vi "Elevator Controller.vi"(8 "error in":errorcluster) -> ()   [LabVIEW 2017]
doc: "This VI executes continuously carrying out the current operation and responding to updates or new operations. It will often contain the timing or control code that is difficult to place directly in TeleOp. This VI generally opens all sensors and motors and isolates the rest of the robot code from knowing how the operations are carried out."
uses:
  <vilib>/Rock Robotics/WPI/Framework/Completion Status.ctl
  Elevator Setpoints.ctl
  Elevator Operations.ctl
  <vilib>/Rock Robotics/WPI/Solenoid/WPI_SolenoidChannel.ctl
  <vilib>/Rock Robotics/WPI/ThirdParty/Phoenix-LabVIEW/Motor Controller/Controls/CTRE_Phoenix_MotorControl_FeedbackDevice.ctl
  <vilib>/Rock Robotics/SystemInterfaces/DIO/FPGA_DIOChannel.ctl
  <vilib>/Rock Robotics/WPI/SafetyOutput/WPI_SafetyOutputConfigMenu.ctl
  <vilib>/Rock Robotics/WPI/ThirdParty/Phoenix-LabVIEW/Motor Controller/Controls/CTRE_Phoenix_MotorControl_NeutralMode.ctl
  <vilib>/Rock Robotics/WPI/ThirdParty/Phoenix-LabVIEW/Motor Controller/Controls/CTRE_Phoenix_MotorControl_ControlMode.ctl
  <vilib>/Rock Robotics/WPI/Solenoid/WPI_SolenoidValue.ctl
  <vilib>/Rock Robotics/WPI/Solenoid/WPI_SolenoidOpenDouble.vi
  <vilib>/Rock Robotics/WPI/Switch/WPI_SwitchOpenLimit.vi
  Elevator Published Globals.vi
  <vilib>/Rock Robotics/WPI/Solenoid/WPI_SolenoidSetEnum.vi
  <vilib>/Rock Robotics/Network Tables/NT Write Boolean.vi
panel:
  in  "Interactive Values":T1
  out "Current\nCmd":string
  in  "Buttons":cluster{"Execute Cmd":bool, "Abort Cmd":bool}
  out "Command Timing":cluster{"Start Time (ms)":u32, "Iterations":i32}
  out "Status":T3
  # "Tip: It may be helpful to observe inputs and sensor values.\nYou may also want to display tuning or debugging controls."
  # "Interactive Command: You may fill in the settings for a command\nand schedule it with the Execute button. You can observe and abort\nany command while fine tuning the code for the controller."
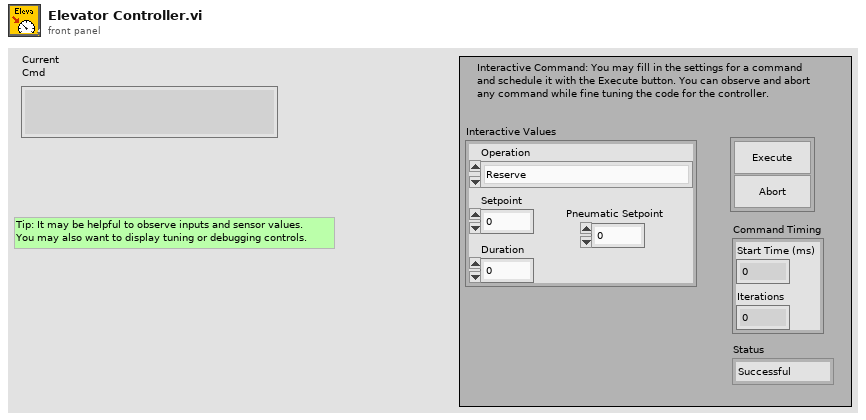
[diagram p1: front panel]
types:
  T1 = typedef "Elevator Setpoints.ctl" = cluster{"Operation":T2, "Setpoint":dbl, "Duration":dbl, "Pneumatic Setpoint":dbl}
  T2 = typedef "Elevator Operations.ctl" = enum16{"Reserve", "Read Current", "Pick Up Cube (Lowest)", "Switch", "Scale", "Immediate"}
  T3 = typedef "Completion Status.ctl" = enum16{"Successful", "Aborted", "Incomplete"}
  T4 = typedef "CTRE_Phoenix_MotorControl_NeutralMode.ctl" = enum8{"EEPROMSetting", "Override to Coast", "Override to Brake"}
  T5 = typedef "WPI_SafetyOutputConfigMenu.ctl" = enum16{"Enable", "Disable"}
  T6 = typedef "FPGA_DIOChannel.ctl" = enum8{"DIO 0", "DIO 1", "DIO 2", "DIO 3", "DIO 4", "DIO 5", "DIO 6", "DIO 7", "DIO 8", "DIO 9", "DIO MXP 0", "DIO MXP 1", "DIO MXP 2", "DIO MXP 3", "DIO MXP 4", "DIO MXP 5", "DIO MXP 6", "DIO MXP 7", "DIO MXP 8", "DIO MXP 9", "DIO MXP 10", "DIO MXP 11", "DIO MXP 12", "DIO MXP 13", "DIO MXP 14", "DIO MXP 15", "SPI Port CS1", "SPI Port CS2", "SPI Port CS3", "SPI Port MISO", "SPI Port MOSI", "Invalid"}
  T7 = typedef "CTRE_Phoenix_MotorControl_FeedbackDevice.ctl" = i8
  T8 = typedef "WPI_SolenoidChannel.ctl" = enum8{"Solenoid 0", "Solenoid 1", "Solenoid 2", "Solenoid 3", "Solenoid 4", "Solenoid 5", "Solenoid 6", "Solenoid 7", "Invalid"}
  T9 = typedef "WPI_MotorControlDeviceRef.ctl" = cluster{"DeviceStatus":errorcluster, "Type":T10, "PWM":cluster{"PWM Channel":T11, "DeadBand":T12}, "CAN":cluster{"Device Number":u8, "SetOutput VI Ref":variant, "GetOutput VI Ref":variant, "Enable VI Ref":variant, "Disable VI Ref":variant, "Data":variant}, "Invert":bool, "DIO PWM":cluster{"PWM \"Enable\" Channel":T11, "DIOChannel":T6, "PWM Rate":dbl}}
  T10 = typedef "WPI_MotorControlType.ctl" = enum16{"PWM", "CAN", "DIO PWM"}
  T11 = typedef "FPGA_DIOPWMChannel.ctl" = enum8{"PWM 0", "PWM 1", "PWM 2", "PWM 3", "PWM 4", "PWM 5", "PWM 6", "PWM 7", "PWM 8", "PWM 9", "PWM MXP 0", "PWM MXP 1", "PWM MXP 2", "PWM MXP 3", "PWM MXP 4", "PWM MXP 5", "PWM MXP 6", "PWM MXP 7", "PWM MXP 8", "PWM MXP 9", "Invalid"}
  T12 = typedef "WPI_PWMDeadband.ctl" = cluster{"Name":string, "maxPositivePwm":i32, "minPositivePwm":i32, "centerPwm":i32, "maxNegativePwm":i32, "minNegativePwm":i32, "angularRange":u16}
  T13 = typedef "WPI_SolenoidDevRef.ctl" = cluster{"DevStatus":errorcluster, "Pneumatics Control Module":u8, "Forward Solenoid Channel":T8, "Reverse Solenoid Channel":T8}
  T14 = typedef "WPI_SwitchDevRef.ctl" = cluster{"DevStatus":errorcluster, "DIO Channel":T6, "CntIndex":T15, "Normally Closed":bool}
  T15 = typedef "FPGA_CounterCtrSystemIndex.ctl" = enum8{"Ctr 0", "Ctr 1", "Ctr 2", "Ctr 3", "Ctr 4", "Ctr 5", "Ctr 6", "Ctr 7", "Invalid"}
  T16 = typedef "Command Status Info.ctl" = cluster{"Name":string, "Status":T3, "notifier out":T17}
  T17 = typedef "Completion Notifier.ctl" = refnum<notifier>
  T18 = cluster{"Current Command":T1, "Command Timing":cluster{"Start Time (ms)":u32, "Iterations":i32}, "Command Arguments":cluster{"Command Info":T16, "Description":string, "Default Command":T1, "queue out":refnum<queue>, "Subsystem Name":string}}
  T19 = typedef "WPI_SolenoidValue.ctl" = enum16{"Off", "On", "Forward", "Reverse"}
  T20 = typedef "CTRE_Phoenix_MotorControl_ControlMode.ctl" = u16
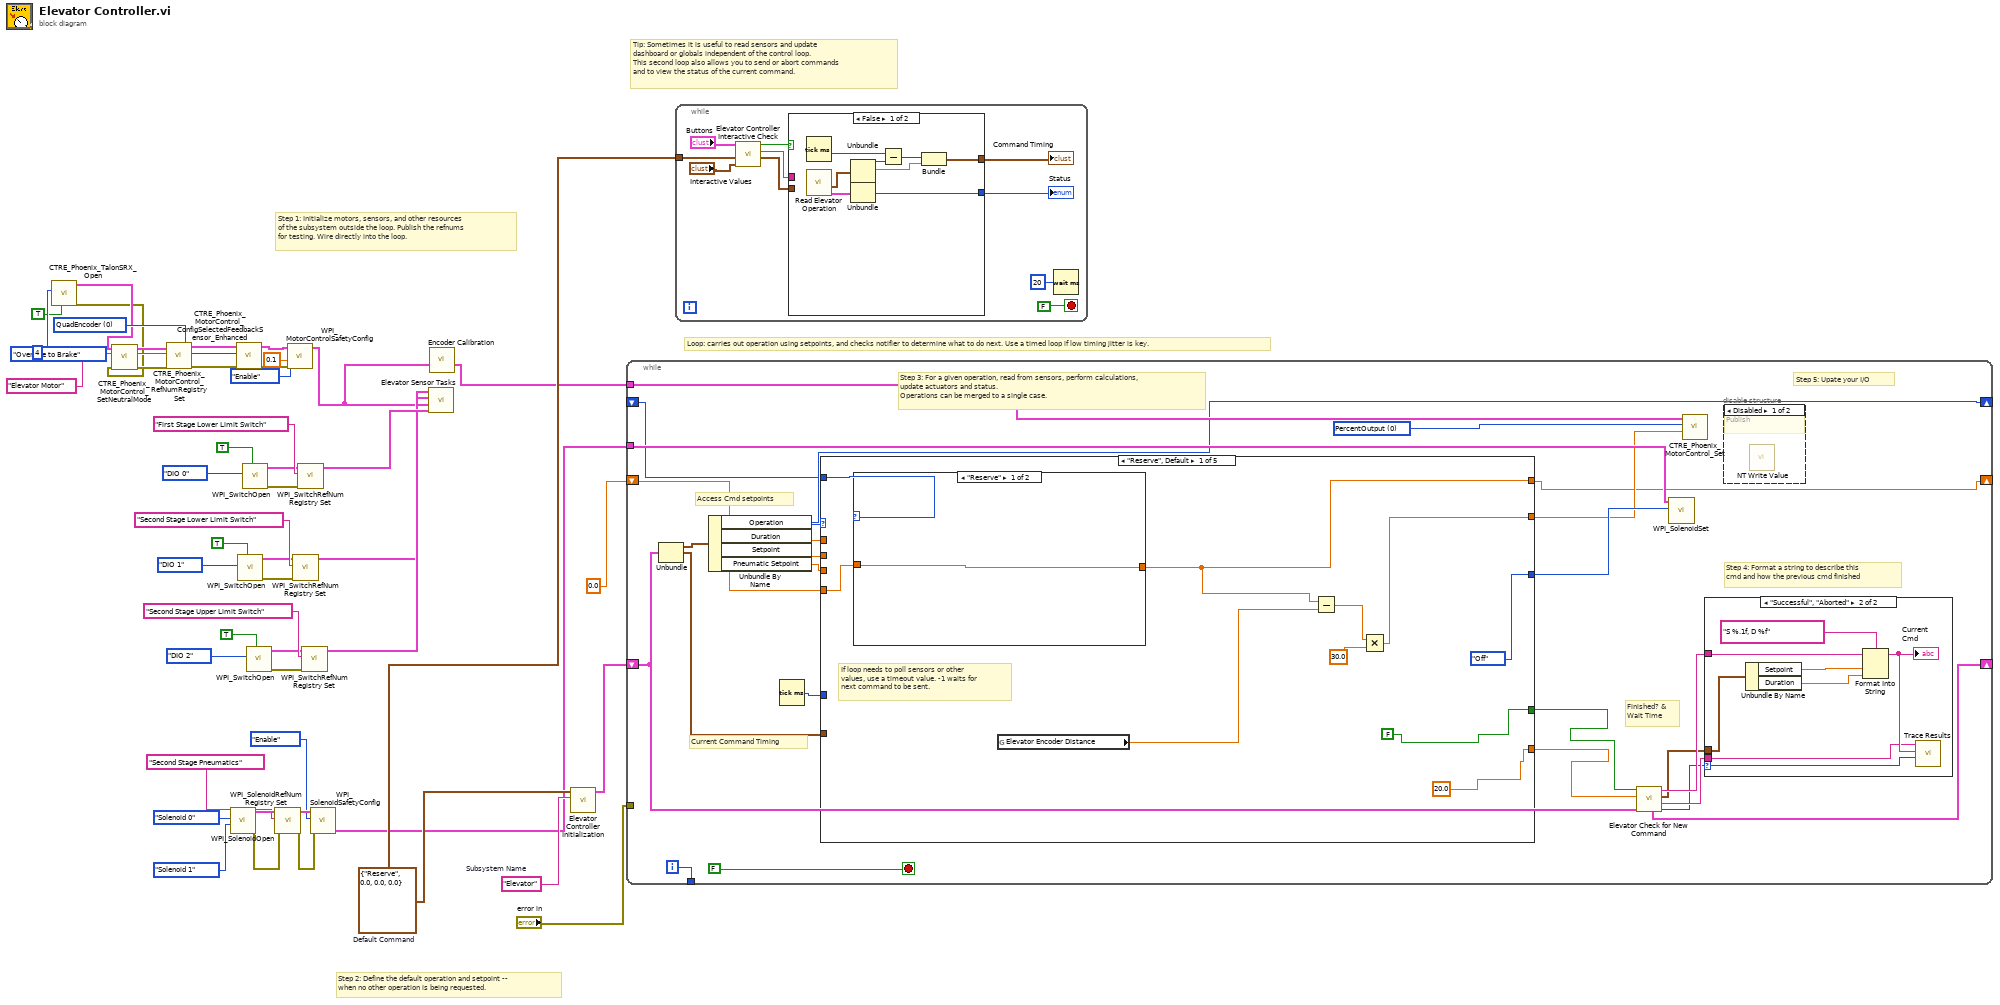
[diagram p0: block diagram]
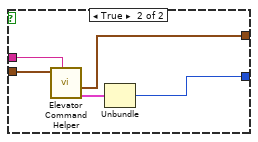
[diagram p2: hidden frame]
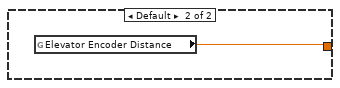
[diagram p5: hidden frame]
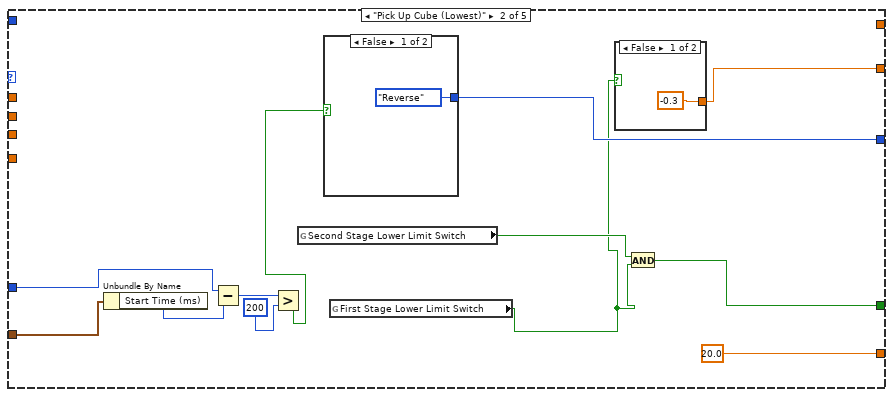
[diagram p6: hidden frame]
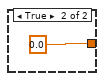
[diagram p7: hidden frame]
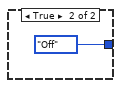
[diagram p8: hidden frame]
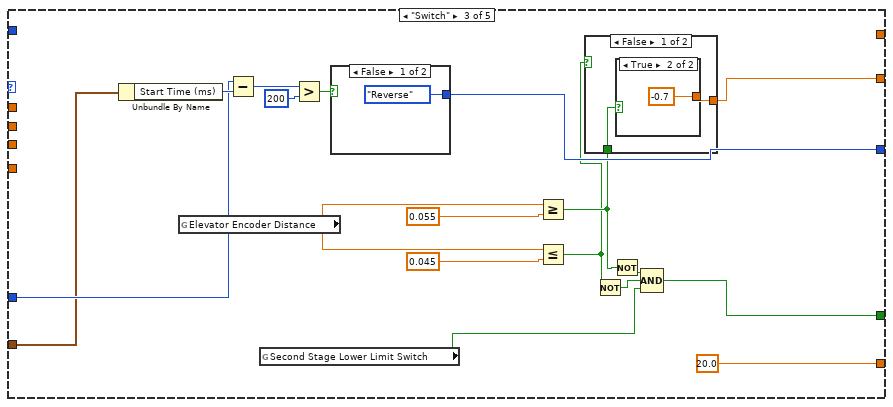
[diagram p9: hidden frame]
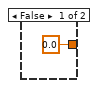
[diagram p10: hidden frame]
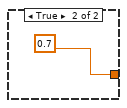
[diagram p11: hidden frame]
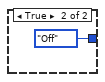
[diagram p12: hidden frame]
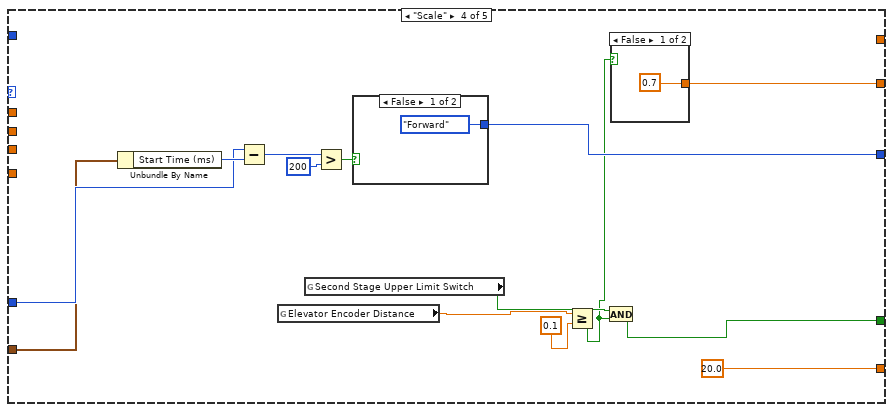
[diagram p13: hidden frame]
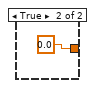
[diagram p14: hidden frame]
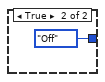
[diagram p15: hidden frame]
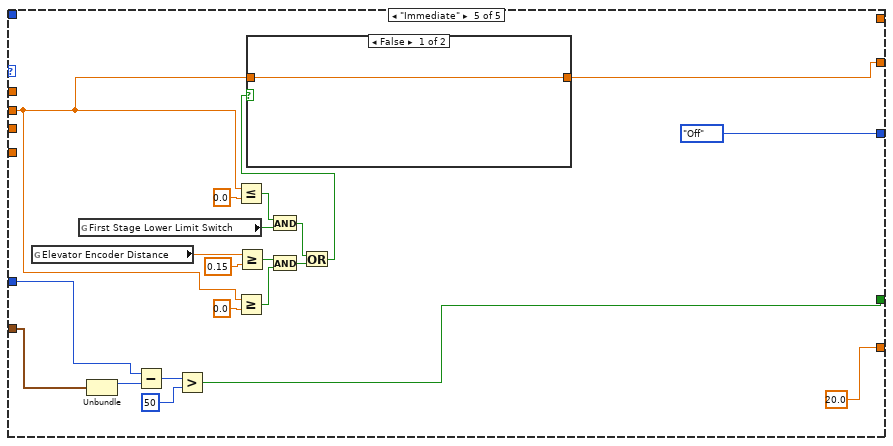
[diagram p16: hidden frame]
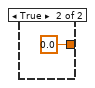
[diagram p17: hidden frame]
diagram:
  w33 = T7 0 items=["None"=-1, "QuadEncoder"=0, "Analog"=2, "Tachometer"=4, "Pulse Width Encoded Position"=8, "Sensor Sum (S0 + S1)"=9, "Sensor Difference (D0 - D1)"=10, "Remote Source 0"=11, "Remote Source 1"=12, "Software Emulated"=15] ("Feedback Device")
  w46 = T1 {"Operation"=enum."Reserve", "Setpoint"=0.0, "Duration"=0.0, "Pneumatic Setpoint"=0.0}  # Default Command
  w47 = "Elevator"  # Subsystem Name
  # "Tip: Sometimes it is useful to read sensors and update\ndashboard or globals independent of the control loop.\nThis second loop also allows you to send or abort commands\nand to view the status of the current command."
  # "Step 2: Define the default operation and setpoint --\nwhen no other operation is being requested."
  # "Step 1: Initialize motors, sensors, and other resources\nof the subsystem outside the loop. Publish the refnums\nfor testing. Wire directly into the loop."
  # "Loop: carries out operation using setpoints, and checks notifier to determine what to do next. Use a timed loop if low timing jitter is key."
  n1 = call <vilib>:"CTRE_Phoenix_TalonSRX_Open.vi"("Invert"=TRUE, "Device Number"=u8 4) -> ("error out"=w22:errorcluster, "CAN Talon SRX Ref"=w25:T9)  [unwired: 8 in]
  n2 = call <vilib>:"CTRE_Phoenix_MotorControl_SetNeutralMode.vi"("error in (no error)"=w22, "Motor Control Neutral Mode"=CTRE_Phoenix_MotorControl_NeutralMode."Override to Brake", "PhoenixMotorControlDevRef"=w25) -> ("error out"=w23:errorcluster, "PhoenixMotorControlDevRef"=w24:T9)  [unwired: 7 in]
  n3 = call <vilib>:"CTRE_Phoenix_MotorControl_RefNumRegistrySet.vi"("error in (no error)"=w23, "refnum name"="Elevator Motor", "PhoenixMotorControlDevRef"=w24) -> ("error out"=w32:errorcluster, "PhoenixMotorControlDevRef"=w34:T9)  [unwired: 7 in]
  n4 = call-poly <vilib>:"WPI_SolenoidOpen.vi"("Reverse Solenoid Channel"=WPI_SolenoidChannel."Solenoid 1", "Forward Solenoid Channel"=WPI_SolenoidChannel."Solenoid 0") -> ("error out"=w42:errorcluster, "SolenoidDevRef"=w43:T13)  [unwired: 8 in]
  n5 = call <vilib>:"CTRE_Phoenix_MotorControl_ConfigSelectedFeedbackSensor_Enhanced.vi"("error in (no error)"=w32, "Feedback Device"=w33, "PhoenixMotorControlDevRef"=w34) -> ("error out"=w5:errorcluster, "PhoenixMotorControlDevRef"=w7:T9)  [unwired: 7 in]
  n6 = call-poly <vilib>:"WPI_SwitchOpen.vi"("Normally Closed"=TRUE, "DIO Channel"=FPGA_DIOChannel."DIO 1") -> ("error out"=w19:errorcluster, "SwitchDevRef"=w17:T14)  [unwired: 8 in]
  n7 = call-poly <vilib>:"WPI_SwitchOpen.vi"("Normally Closed"=TRUE, "DIO Channel"=FPGA_DIOChannel."DIO 0") -> ("error out"=w29:errorcluster, "SwitchDevRef"=w27:T14)  [unwired: 8 in]
  n8 = call-poly <vilib>:"WPI_SwitchOpen.vi"("Normally Closed"=TRUE, "DIO Channel"=FPGA_DIOChannel."DIO 2") -> ("error out"=w14:errorcluster, "SwitchDevRef"=w12:T14)  [unwired: 8 in]
  n9 = call <vilib>:"WPI_SolenoidRefNum Registry Set.vi"("error in (no error)"=w42, "refnum name"="Second Stage Pneumatics", "SolenoidDevRef"=w43) -> ("error out"=w41:errorcluster, "SolenoidDevRef"=w44:T13)  [unwired: 7 in]
  n10 = call <vilib>:"WPI_MotorControlSafetyConfig.vi"("error in (no error)"=w5, "timeout (s)"=0.1, "mode"=WPI_SafetyOutputConfigMenu."Enable", "MotorControlDevRef"=w7) -> ("MotorControlDevRef"=w6:T9)  [unwired: 6 in, 1 out]
  n11 = call <vilib>:"WPI_SwitchRefNum Registry Set.vi"("error in (no error)"=w19, "refnum name"="Second Stage Lower Limit Switch", "SwitchDevRef"=w17) -> ("SwitchDevRef"=w10:T14)  [unwired: 7 in, 1 out]
  n12 = call <vilib>:"WPI_SwitchRefNum Registry Set.vi"("error in (no error)"=w29, "refnum name"="First Stage Lower Limit Switch", "SwitchDevRef"=w27) -> ("SwitchDevRef"=w26:T14)  [unwired: 7 in, 1 out]
  n13 = call <vilib>:"WPI_SwitchRefNum Registry Set.vi"("error in (no error)"=w14, "refnum name"="Second Stage Upper Limit Switch", "SwitchDevRef"=w12) -> ("SwitchDevRef"=w11:T14)  [unwired: 7 in, 1 out]
  n14 = call <vilib>:"WPI_SolenoidSafetyConfig.vi"("error in (no error)"=w41, "mode"=WPI_SafetyOutputConfigMenu."Enable", "SolenoidDevRef"=w44) -> ("SolenoidDevRef"=w45:T13)  [unwired: 7 in, 1 out]
  n15 = call "Elevator Sensor Tasks.vi"("SecondUpperElevatorSwitchDevRef"=w11, "SecondLowerElevatorSwitchDevRef"=w10, "ElevatorControllerDevRef"=w6, "FirstLowerElevatorSwitchDevRef"=w26) -> ()  [unwired: 7 in]
  n16 = call "Encoder Calibration.vi"("PhoenixMotorControlDevRef"=w6) -> ("PhoenixMotorControlDevRef Out"=w9:T9)  [unwired: 10 in]
  n17 = call "Elevator Controller Initialization.vi"("Subsystem Name"=w47, "Default Command"=w46) -> ("Current Command"=w48:T18)  [unwired: 9 in]
  n18 = while {
    shift-right: [w67] -> _
    shift-left: w48 -> [w60]
    tunnel: [w73] -> _
    tunnel: "error in" -> [_]
    tunnel: w45 -> [w59]
    tunnel: w9 -> [w57]
    shift-right: [w53] -> _
    shift-left: _ -> [w52]
    shift-right: [w51] -> _
    shift-left: 0.0 -> [w50]
    i -> [w73]
    stop <- FALSE stop-if-true
    w56 = T20 0 items=["PercentOutput"=0, "Position"=1, "Velocity"=2, "Current"=3, "Follower"=5, "MotionProfile"=6, "MotionMagic"=7, "MotionMagicArc"=8, "MotionProfileArc"=10, "Disabled"=15] ("Control Mode")
    # "Step 5: Upate your I/O"
    # "Step 4: Format a string to describe this\ncmd and how the previous cmd finished"
    # "Current Command Timing"
    # "Access Cmd setpoints"
    # "Finished? &\nWait Time"
    # "Step 3: For a given operation, read from sensors, perform calculations,\nupdate actuators and status.\nOperations can be merged to a single case."
    n19 = Unbundle(w60) -> ("Current Command"=w72:T1, "Command Timing"=w69:cluster{"Start Time (ms)":u32, "Iterations":i32})  [unwired: 1 out]
    n20 = Unbundle By Name(w72) -> ("Operation"=w53:T2, "Duration"=w71:dbl, "Setpoint"=w68:dbl, "Pneumatic Setpoint"=w58:dbl)
    n21 = Tick Count (ms)() -> (millisecond timer value=w70:u32)
    n22 = case shown="\"Reserve\", Default" w53 {
      tunnel: [20.0 20.0 ("Infinite") 20.0 ("Infinite") 20.0 ("Infinite") 20.0 ("Infinite")] -> w65
      tunnel: [FALSE ("First Stage Lower Limit Switch") w97 w115 w138 w167] -> w66
      tunnel: w69 -> [_ w99 w121 w144 w168]
      tunnel: w71 -> [_ _ _ _ _]
      tunnel: w70 -> [_ w100 w122 w145 w169]
      tunnel: w68 -> [_ _ _ _ w157]
      tunnel: w58 -> [_ _ _ _ _]
      tunnel: [WPI_SolenoidValue."Off" ("Value") w101 w126 w142 WPI_SolenoidValue."Off" ("Value")] -> w55
      tunnel: [w83 w95 w117 w137 w166] -> w54
      tunnel: w52 -> [w90 _ _ _ _]
      tunnel: [w87 _ _ _ _] -> w51
      tunnel: w50 -> [w89 _ _ _ _]
      frame "Reserve", Default {
        # "If loop needs to poll sensors or other\nvalues, use a timeout value. -1 waits for\nnext command to be sent."
        n23 = case shown="\"Reserve\"" w90 {
          tunnel: [w93 w94] -> w87
          tunnel: w89 -> [w93 _]
          frame "Reserve" {
          }
          frame Default {
            n24 = global read "Elevator Published Globals.vi" "Elevator Encoder Distance"() -> (w94:dbl)
          }
        }
        n25 = global read "Elevator Published Globals.vi" "Elevator Encoder Distance"() -> (w86:dbl)
        n26 = Subtract(x=w87, y=w86) -> (x-y=w85:dbl)
        n27 = Multiply(x=w85, y=30.0) -> (x*y=w83:dbl)
      }
      frame "Pick Up Cube (Lowest)" {
        n28 = Unbundle By Name(w99) -> ("Start Time (ms)"=w105:u32)
        n29 = Subtract(x=w100, y=w105) -> (x-y=w104:u32)
        n30 = Greater?(x=w104, y=u8 200 ("Left Motor")) -> (0:w102:bool)
        n31 = global read "Elevator Published Globals.vi" "Second Stage Lower Limit Switch"() -> (w98:bool)
        n32 = case shown="False" w102 {
          tunnel: [WPI_SolenoidValue."Reverse" ("Value") WPI_SolenoidValue."Off" ("Value")] -> w101
          frame False {
          }
          frame True {
          }
        }
        n33 = global read "Elevator Published Globals.vi" "First Stage Lower Limit Switch"() -> (w96:bool)
        n34 = case shown="False" w96 {
          tunnel: [-0.3 0.0] -> w95
          frame False {
          }
          frame True {
          }
        }
        n35 = And(x=w98, y=w96) -> (x .and. y?=w97:bool)
      }
      frame "Switch" {
        n36 = Unbundle By Name(w121) -> ("Start Time (ms)"=w125:u32)
        n37 = global read "Elevator Published Globals.vi" "Elevator Encoder Distance"() -> (w119:dbl)
        n38 = Subtract(x=w122, y=w125) -> (x-y=w124:u32)
        n39 = global read "Elevator Published Globals.vi" "Second Stage Lower Limit Switch"() -> (w116:bool)
        n40 = Greater?(x=w124, y=u8 200 ("Left Motor")) -> (0:w120:bool)
        n41 = case shown="False" w120 {
          tunnel: [WPI_SolenoidValue."Reverse" ("Value") WPI_SolenoidValue."Off" ("Value")] -> w126
          frame False {
          }
          frame True {
          }
        }
        n42 = Greater Or Equal?(x=w119, y=0.055) -> (x >= y?=w113:bool)
        n43 = Less Or Equal?(x=w119, y=0.045) -> (x <= y?=w112:bool)
        n44 = case shown="False" w112 {
          tunnel: w113 -> [w130 _]
          tunnel: [w129 0.7] -> w117
          frame False {
            n45 = case shown="True" w130 {
              tunnel: [0.0 -0.7] -> w129
              frame False {
              }
              frame True {
              }
            }
          }
          frame True {
          }
        }
        n46 = Not(x=w112) -> (.not. x?=w114:bool)
        n47 = Not(x=w113) -> (.not. x?=w111:bool)
        n48 = Compound Arithmetic op=AND(w111, w114, w116) -> (w115:bool)
      }
      frame "Scale" {
        n49 = Unbundle By Name(w144) -> ("Start Time (ms)"=w148:u32)
        n50 = Subtract(x=w145, y=w148) -> (x-y=w147:u32)
        n51 = global read "Elevator Published Globals.vi" "Elevator Encoder Distance"() -> (w141:dbl)
        n52 = global read "Elevator Published Globals.vi" "Second Stage Upper Limit Switch"() -> (w139:bool)
        n53 = Greater?(x=w147, y=u8 200 ("Left Motor")) -> (0:w143:bool)
        n54 = case shown="False" w143 {
          tunnel: [WPI_SolenoidValue."Forward" ("Value") WPI_SolenoidValue."Off" ("Value")] -> w142
          frame False {
          }
          frame True {
          }
        }
        n55 = Greater Or Equal?(x=w141, y=0.1) -> (x >= y?=w136:bool)
        n56 = And(x=w139, y=w136) -> (x .and. y?=w138:bool)
        n57 = case shown="False" w136 {
          tunnel: [0.7 0.0] -> w137
          frame False {
          }
          frame True {
          }
        }
      }
      frame "Immediate" {
        n58 = global read "Elevator Published Globals.vi" "Elevator Encoder Distance"() -> (w165:dbl)
        n59 = global read "Elevator Published Globals.vi" "First Stage Lower Limit Switch"() -> (w160:bool)
        n60 = Unbundle(w168) -> ("Start Time (ms)"=w170:u32)  [unwired: 1 out]
        n61 = Subtract(x=w169, y=w170) -> (x-y=w171:u32)
        n62 = Greater?(x=w171, y=u8 50 ("Left Motor")) -> (0:w167:bool)
        n63 = Less Or Equal?(x=w157, y=0.0) -> (x <= y?=w161:bool)
        n64 = Greater Or Equal?(x=w157, y=0.0) -> (x >= y?=w156:bool)
        n65 = Greater Or Equal?(x=w165, y=0.15) -> (x >= y?=w155:bool)
        n66 = And(x=w161, y=w160) -> (x .and. y?=w159:bool)
        n67 = And(x=w155, y=w156) -> (x .and. y?=w154:bool)
        n68 = Or(x=w159, y=w154) -> (x .or. y?=w164:bool)
        n69 = case shown="False" w164 {
          tunnel: [w175 0.0 ("Setpoint")] -> w166
          tunnel: w157 -> [w175 _]
          frame False {
          }
          frame True {
          }
        }
      }
    }
    n70 = call "Elevator Check for New Command.vi"("Current Command"=w60, "Wait time (ms)"=w65, "Finished?"=w66) -> ("Completion"=w61:T3, "Subsystem Name"=w62:string, "Current Command"=w63:T1, "Initial Trace String"=w64:string, "NextCommand"=w67:T18)  [unwired: 4 in]
    n71 = call-poly <vilib>:"WPI_SolenoidSet.vi"("Value"=w55, "SolenoidDevRef"=w59) -> ()  [unwired: 8 in, 2 out]
    n72 = call <vilib>:"CTRE_Phoenix_MotorControl_Set.vi"("Output"=w54, "Control Mode"=w56, "PhoenixMotorControlDevRef"=w57) -> ()  [unwired: 7 in, 2 out]
    n73 = case shown="\"Successful\", \"Aborted\"" w61 {
      selector: w61 -> [_ w82]
      tunnel: w64 -> [_ w78]
      tunnel: w63 -> [_ w79]
      tunnel: w62 -> [_ w75]
      frame "Incomplete", Default {
        # "Continuing current command"
      }
      frame "Successful", "Aborted" {
        # "Report and setup for next command"
        n74 = Unbundle By Name(w79) -> ("Setpoint"=w81:dbl, "Duration"=w76:dbl)
        n75 = Format Into String(format string="S %.1f, D %f", initial string=w78, w81, w76) -> (resulting string=w77:string)  [unwired: 1 in, 1 out]
        "Current\nCmd" <- w77
        n76 = call <vilib>:"Trace Results.vi"("Status of previous command"=w82, "Description"=w77, "Subsystem"=w75) -> ()  [unwired: 9 in]
      }
    }
    n77 = disable-structure shown="Disabled" {
      frame Disabled {
        # "Publish"
        n78 = call-poly <vilib>:"NT Write Value.vi"() -> ()  [unwired: 11 in, 1 out]
      }
      frame Enabled {
      }
    }
  }
  n79 = while {
    tunnel: w46 -> [w183]
    stop <- FALSE stop-if-true
    n80 = call "Elevator Controller Interactive Check.vi"("Interactive Command in"="Interactive Values", "Default Command"=w183, "Buttons"="Buttons") -> ("Interactive Command out"=w180:T1, "Trace String"=w181:string, "Schedule"=w182:bool)  [unwired: 6 in]
    n81 = case shown="False" w182 {
      tunnel: [w194 w199] -> w179
      tunnel: w180 -> [_ w197]
      tunnel: [w190 w195] -> w178
      tunnel: w181 -> [_ w198]
      frame False {
        n82 = Tick Count (ms)() -> (millisecond timer value=w189:u32)
        n83 = call "Read Elevator Operation.vi"() -> ("Command Info"=w187:T16, "SubSystem Data"=w188:T1)  [unwired: 9 in, 1 out]
        n84 = Unbundle(w188) -> ("Operation"=w193:T2, "Setpoint"=w191:dbl)  [unwired: 2 out]
        n85 = Unbundle(w187) -> ("Status"=w194:T3)  [unwired: 2 out]
        n86 = Subtract(x=w189, y=w193) -> (x-y=w192:u32)
        n87 = Bundle(w192, "Setpoint"=w191) -> (w190:cluster{u32, "Setpoint":dbl})  [unwired: 1 in]
      }
      frame True {
        n88 = call "Elevator Command Helper.vi"("Description"=w198, "SubSystem Data"=w197) -> ("Command Info Out"=w196:T16, "Command Timing"=w195:cluster{"Start Time (ms)":u32, "Iterations":i32})  [unwired: 7 in, 1 out]
        n89 = Unbundle(w196) -> ("Status"=w199:T3)  [unwired: 2 out]
      }
    }
    "Status" <- w179
    "Command Timing" <- w178
    n90 = Wait (ms)(milliseconds to wait=u32 20) -> ()  [unwired: 1 out]
  }
